vi "Star shape.vi"(8 "error in":errorcluster, 11 "Size":enum16{"Small", "Medium", "Large"}(ring)) -> (0 "error out":errorcluster, 3 "XY Graph":cluster{"X coords":dbl[], "Y coords":dbl[]}(graph))   [LabVIEW 2017]
doc: "To draw a star shape on the spherical object with with different sizes (small, medium and large)."
panel:
  out "dy":i32[](array[numeric])
  out "dx":i32[](array[numeric])
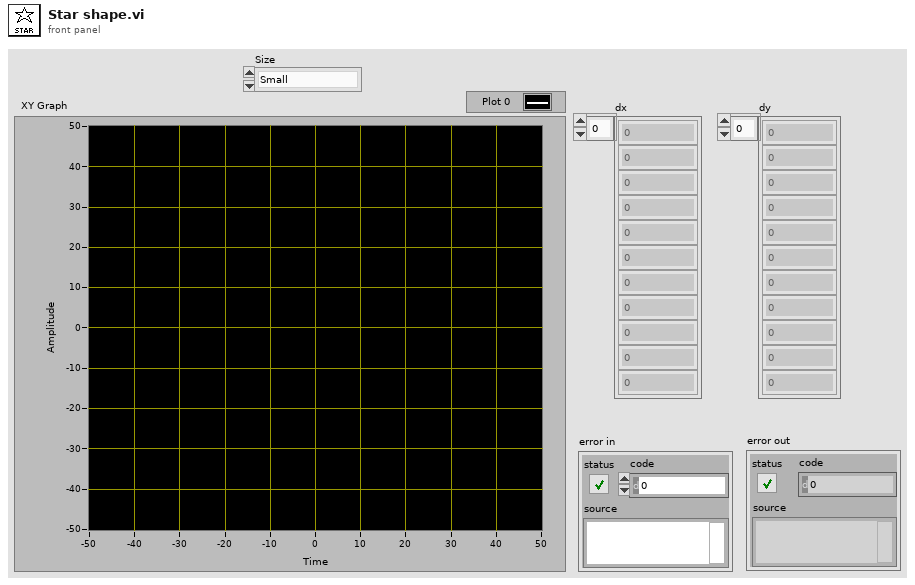
[diagram p1: front panel]
types:
  T1 = enum16{"Full", "Half", "Quarter", "Eighth", "Sixteenth"}
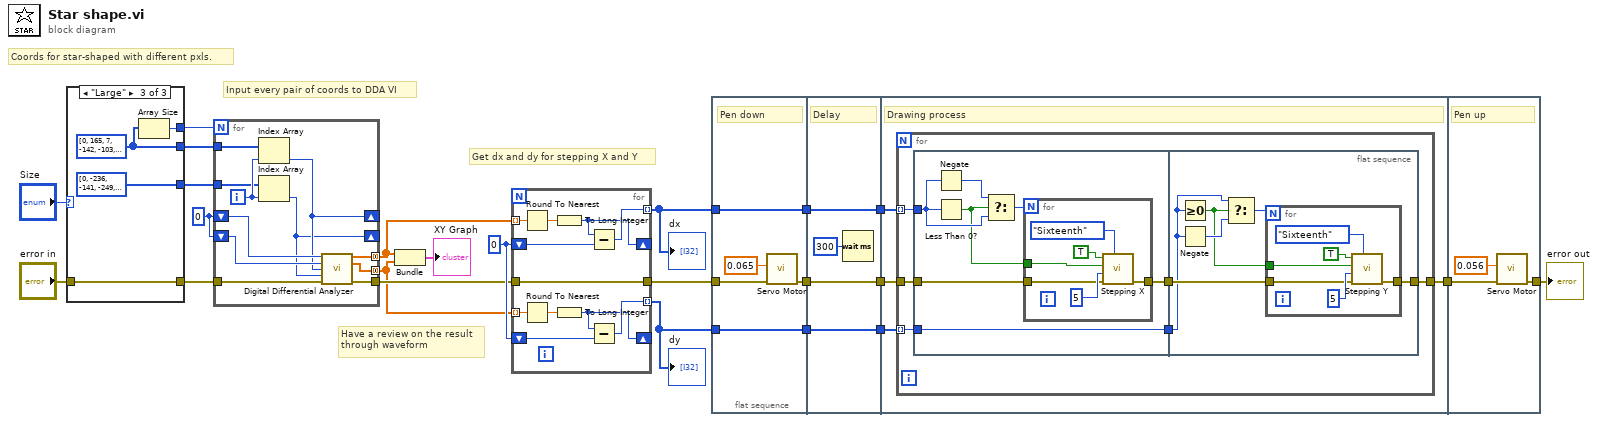
[diagram p0: block diagram]
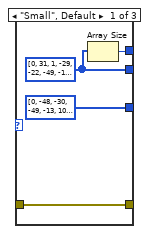
[diagram p2: hidden frame]
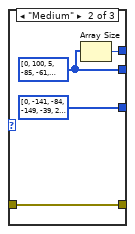
[diagram p3: hidden frame]
diagram:
  w7 = 0 ("Numeric")
  w23 = 0
  # "Have a review on the result\nthrough waveform"
  # "Input every pair of coords to DDA VI"
  # "Coords for star-shaped with different pxls."
  # "Get dx and dy for stepping X and Y"
  n1 = case shown="\"Large\"" "Size" {
    tunnel: [w26 w30 w34] -> w20
    tunnel: [w25 w29 w33] -> w19
    tunnel: [i32[] [0, -48, -30, -49, -13, 10, 15, 49, 15, 13, -12, -48] ("Y (100 pxl)") i32[] [0, -141, -84, -149, -39, 29, 40, 147, 44, 42, -33, -141] ("Y (300 pxl)") i32[] [0, -236, -141, -249, -65, 48, 67, 245, 73, 69, -56, -236] ("Y (500 pxl)")] -> w18
    tunnel: "error in" -> [w24 w28 w32]
    tunnel: [w24 w28 w32] -> w17
    frame "Small", Default {
      w25 = i32[] [0, 31, 1, -29, -22, -49, -14, -1, 14, 49, 23, 31] ("X (100 pxl)")
      n2 = Array Size(array=w25) -> (size(s)=w26:i32)
    }
    frame "Medium" {
      w29 = i32[] [0, 100, 5, -85, -61, -149, -40, -4, 40, 150, 68, 100] ("X (300 pxl)")
      n3 = Array Size(array=w29) -> (size(s)=w30:i32)
    }
    frame "Large" {
      w33 = i32[] [0, 165, 7, -142, -103, -249, -68, -8, 65, 248, 112, 165] ("X (500 pxl)")
      n4 = Array Size(array=w33) -> (size(s)=w34:i32)
    }
  }
  n5 = for {
    N: w20 -> [_]
    shift-right: [w43] -> _
    shift-left: w7 -> [w45]
    shift-right: [w42] -> _
    shift-left: w7 -> [w44]
    tunnel: [w40] -> w11 mode=concatenating
    tunnel: [w41] -> w10 mode=concatenating
    tunnel: w19 -> [w39]
    tunnel: w18 -> [w38]
    tunnel: w17 -> [w37]
    tunnel: [w36] -> w15
    i -> [w46]
    n6 = Index Array(array=w39, index=w46) -> (element=w43:i32)
    n7 = Index Array(array=w38, index=w46) -> (element=w42:i32)
    n8 = call "Digital Differential Analyzer.vi"("x0"=w45, "y0"=w44, "x1"=w43, "y1"=w42, "error in (no error)"=w37) -> ("X coords"=w40:dbl[], "Y coords"=w41:dbl[], "error out"=w36:errorcluster)  [unwired: 8 in]
  }
  n9 = Bundle("X coords"=w11, "Y coords"=w10) -> (→"XY Graph":cluster{"X coords":dbl[], "Y coords":dbl[]})  [unwired: 1 in]
  n10 = for {
    shift-right: [w51] -> _
    shift-left: w23 -> [w57]
    shift-right: [w50] -> _
    shift-left: w23 -> [w55]
    tunnel: w11 -> [w53] mode=indexing
    tunnel: w10 -> [w52] mode=indexing
    tunnel: [w56] -> w22 mode=indexing
    tunnel: [w54] -> w8 mode=indexing
    tunnel: w15 -> [w47]
    tunnel: [w47] -> w14
    n11 = Round To Nearest(number=w53) -> (nearest integer value=w49:dbl)
    n12 = Round To Nearest(number=w52) -> (nearest integer value=w48:dbl)
    n13 = To Long Integer(number=w49) -> (32bit integer=w51:i32)
    n14 = To Long Integer(number=w48) -> (32bit integer=w50:i32)
    n15 = Subtract(x=w51, y=w57) -> (x-y=w56:i32)
    n16 = Subtract(x=w50, y=w55) -> (x-y=w54:i32)
  }
  "dx" <- w22
  "dy" <- w8
  n17 = flat-sequence {
    tunnel: w8 -> [w61]
    tunnel: w22 -> [w62]
    tunnel: [w62] -> w6
    tunnel: [w61] -> w4
    tunnel: w14 -> [w59]
    tunnel: [w58] -> w2
    tunnel: w6 -> [w66]
    tunnel: [w66] -> w5
    tunnel: w4 -> [w65]
    tunnel: [w65] -> w3
    tunnel: w2 -> [w64]
    tunnel: [w64] -> w1
    tunnel: w5 -> [w70]
    tunnel: w3 -> [w69]
    tunnel: w1 -> [w68]
    tunnel: [w67] -> w13
    tunnel: w13 -> [w103]
    tunnel: [w102] -> w12
    frame #0 {
      # "Pen down"
      n18 = call "Servo Motor.vi"("error in (no error)"=w59, "Duty Cycle"=0.065) -> ("error out"=w58:errorcluster)  [unwired: 9 in]
    }
    frame #1 {
      # "Delay"
      n19 = Wait (ms)(milliseconds to wait=u32 300) -> ()  [unwired: 1 out]
    }
    frame #2 {
      # "Drawing process"
      n20 = for {
        tunnel: w70 -> [w76] mode=indexing
        tunnel: w69 -> [w71] mode=indexing
        tunnel: w68 -> [w75]
        tunnel: [w73] -> w67
        n21 = flat-sequence {
          tunnel: w76 -> [w82]
          tunnel: w75 -> [w79]
          tunnel: [w78] -> w74
          tunnel: [w77] -> w72
          tunnel: w71 -> [w77]
          tunnel: w74 -> [w92]
          tunnel: [w91] -> w73
          tunnel: w72 -> [w90]
          frame #0 {
            n22 = Negate(x=w82) -> (-x=w83:i32)
            n23 = Less Than 0?(x=w82) -> (x < 0?=w81:bool)
            n24 = Select(t=w83, s=w81, f=w82) -> (s? t:f=w80:i32)
            n25 = for {
              N: w80 -> [_]
              tunnel: w81 -> [w86]
              tunnel: w79 -> [w85]
              tunnel: [w84] -> w78
              n26 = call "Stepping X.vi"("Microstep size"=T1."Sixteenth", "error in (no error)"=w85, "Delay"=u32 5 ("Speed"), "Direction"=w86, "Enable"=TRUE) -> ("error out"=w84:errorcluster)  [unwired: 6 in]
            }
          }
          frame #1 {
            n27 = Greater Or Equal To 0?(x=w90) -> (x >= 0?=w93:bool)
            n28 = Negate(x=w90) -> (-x=w95:i32)
            n29 = Select(t=w90, s=w93, f=w95) -> (s? t:f=w94:i32)
            n30 = for {
              N: w94 -> [_]
              tunnel: w93 -> [w98]
              tunnel: w92 -> [w97]
              tunnel: [w96] -> w91
              n31 = call "Stepping Y.vi"("Microstep size"=T1."Sixteenth", "error in (no error)"=w97, "Delay"=u32 5 ("Speed"), "Direction"=w98, "Enable"=TRUE) -> ("error out"=w96:errorcluster)  [unwired: 6 in]
            }
          }
        }
      }
    }
    frame #3 {
      # "Pen up"
      n32 = call "Servo Motor.vi"("error in (no error)"=w103, "Duty Cycle"=0.056) -> ("error out"=w102:errorcluster)  [unwired: 9 in]
    }
  }
  "error out" <- w12
